vi "Example_pico_data_acquisition_tool.vi"() -> ()   [LabVIEW 2022 SP3]
uses:
  usbtmc_scpi_labtool.lvlib
panel:
  out "Meter":dbl(knob) scale=-4.0..4.0 scale format="%#_6f"
  in  "ID Query (True)":bool=TRUE
  in  "ID query string":string="PICO-PI,ANALOGTOOL"
  out "voltage out":dbl format="%#_5f"
  in  "Pin":u8 max=1 step=1
  in  "stop":bool
  in  "VISA resource name in":refnum<visa-resource-name>
  # "For this example, load the analogtool firmware\nhttps://github.com/jancumps/pico_scpi_usbtms_analogtool"
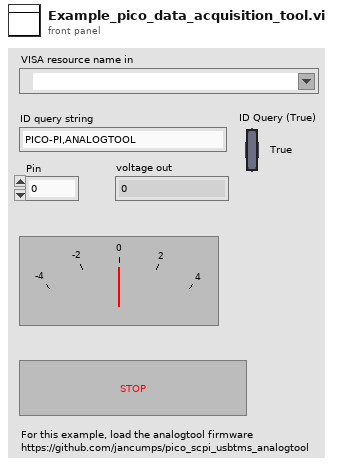
[diagram p1: front panel]
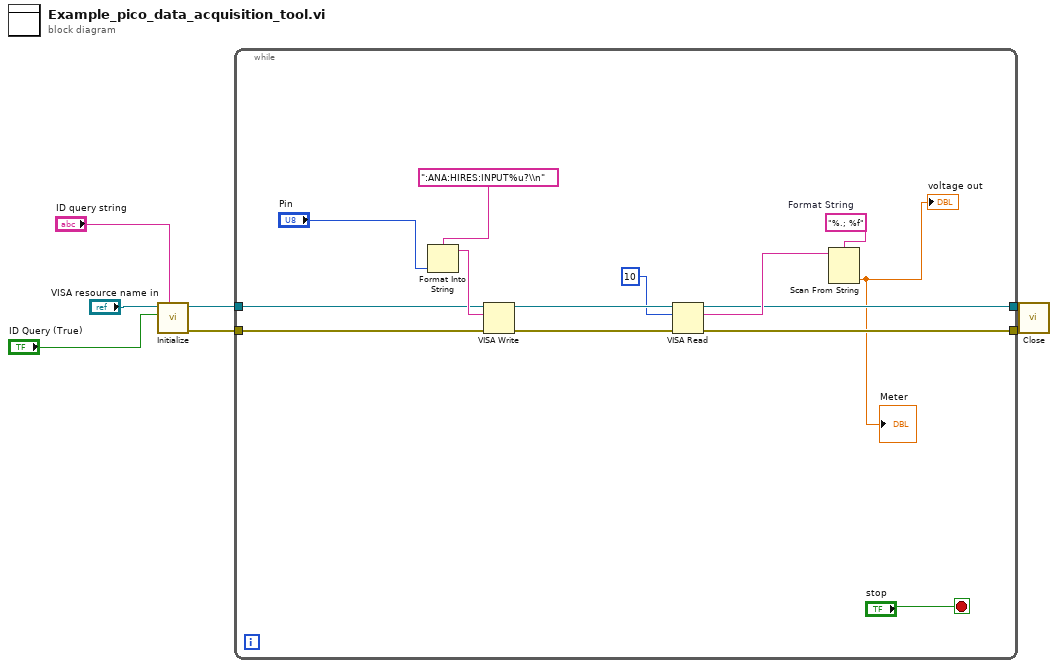
[diagram p0: block diagram]
diagram:
  n1 = call "Initialize.vi"("ID query string"="ID query string", "ID Query (True)"="ID Query (True)", "VISA resource name in"="VISA resource name in") -> ("error out"=w6:errorcluster, "VISA resource name out"=w7:refnum<visa-resource-name>)  [unwired: 7 in]
  n2 = while {
    tunnel: w7 -> [w12]
    tunnel: [w9] -> w5
    tunnel: w6 -> [w11]
    tunnel: [w10] -> w4
    stop <- "stop" stop-if-true
    w16 = "%.; %f"  # Format String
    n3 = Format Into String(format string=":ANA:HIRES:INPUT%u?\\n", "Pin") -> (resulting string=w17:string)  [unwired: 2 in, 1 out]
    n4 = VISA Write(VISA resource name=w12, write buffer=w17, error in (no error)=w11) -> (VISA resource name out=w19:refnum<visa-resource-name>, error out=w20:errorcluster)  [unwired: 1 out]
    n5 = VISA Read(VISA resource name=w19, byte count=u32 10, error in (no error)=w20) -> (VISA resource name out=w9:refnum<visa-resource-name>, read buffer=w18:string, error out=w10:errorcluster)  [unwired: 1 out]
    n6 = Scan From String(format string=w16, input string=w18) -> (output 1=→"voltage out" →"Meter":dbl)  [unwired: 3 in, 3 out]
  }
  n7 = call "Close.vi"("error in (no error)"=w4, "VISA resource name"=w5) -> ()  [unwired: 10 in]
